vi "Custom Event Response.vi"(8 "error in (no error)":errorcluster, 9 "Data":variant, 10 "Cmd":string, 11 "Connector Editor Handler in":refnum<class "Connector Editor Handler.lvclass">) -> (0 "error out":errorcluster, 3 "Connector Editor Handler out":refnum<class "Connector Editor Handler.lvclass">)   [LabVIEW 2017, in "Connector Editor Handler.lvclass"]
uses:
  Connector Editor Handler.lvclass
  Connector Editor Handler.lvclass/Connector Editor Handler.ctl
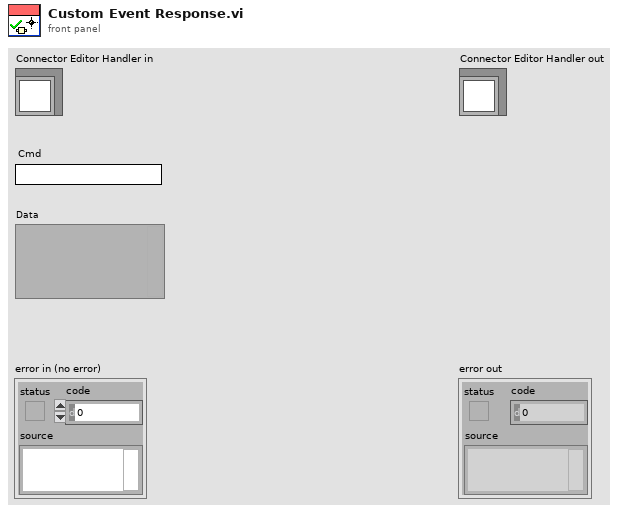
[diagram p1: front panel]
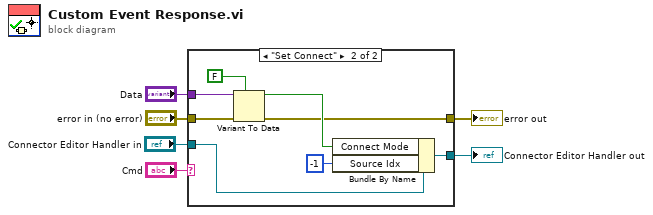
[diagram p0: block diagram]
diagram:
  n1 = case shown="\"Set Connect\"" "Cmd" {
    tunnel: "Connector Editor Handler in" -> [w7 w16]
    tunnel: "Data" -> [_ w15]
    tunnel: "error in (no error)" -> [w8 w12]
    tunnel: [w8 w11] -> w2
    tunnel: [w7 w10] -> w1
    frame Default {
    }
    frame "Set Connect" {
      n2 = Variant To Data(error in=w12, type=FALSE, Variant=w15) -> (data=w13:bool, error out=w11:errorcluster)
      n3 = Bundle By Name(cluster=w16, "Connect Mode"=w13, "Source Idx"=-1) -> (w10:refnum<class "Connector Editor Handler.lvclass">)
    }
  }
  "error out" <- w2
  "Connector Editor Handler out" <- w1
